vi "RPC Method Measurement_v1_MeasurementService_Measure.vi"(8 "error in (no error)":errorcluster, 10 "Request Data":T4, 11 "gRPC Client in":refnum<class "Measurement_lv_client.lvclass">) -> (0 "error out":errorcluster, 2 "Response Data":T1, 3 "gRPC Client out":refnum<class "Measurement_lv_client.lvclass">)   [LabVIEW 2020, in "Measurement_lv_client.lvlib" / "Measurement_lv_client.lvclass"]
uses:
  Measurement_lv_client.lvclass
  RPC Messages/Measurement_v1_MeasureRequest/Measurement_v1_MeasureRequest_Data.ctl
  RPC Messages/google_protobuf_Any/google_protobuf_Any_Data.ctl
  RPC Messages/Measurement_v1_MeasureResponse/Measurement_v1_MeasureResponse_Data.ctl
  RPC Messages/Measurement_v1_ErrorInformation/Measurement_v1_ErrorInformation_Data.ctl
  Measurement_lv_client.lvclass/Measurement_lv_client.ctl
  fa22ca14-33b2-4bc3-8699-3f27c9b27c9c.vi
  <vilib>/gRPC/LabVIEW gRPC Library/Server API/Server/Get Server DLL Path.vi
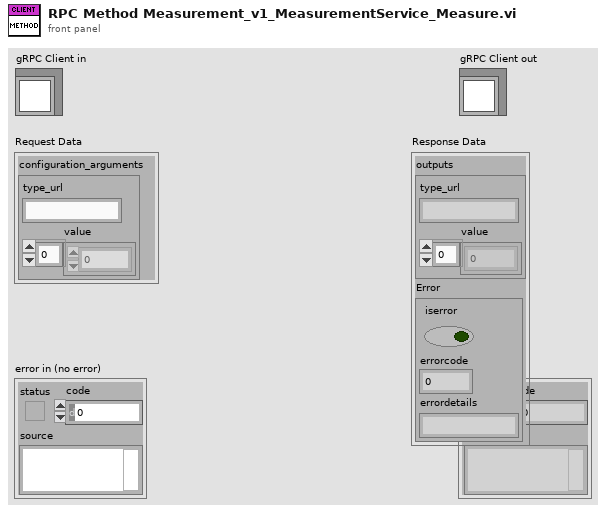
[diagram p1: front panel]
types:
  T1 = typedef "Measurement_lv_client.lvlib/Measurement_lv_client.lvclass/Measurement_v1_MeasureResponse_Data.ctl" = cluster{"outputs":T2, "Error":T3}
  T2 = typedef "Measurement_lv_client.lvlib/Measurement_lv_client.lvclass/google_protobuf_Any_Data.ctl" = cluster{"type_url":string, "value":u8[]}
  T3 = typedef "Measurement_lv_client.lvlib/Measurement_lv_client.lvclass/Measurement_v1_ErrorInformation_Data.ctl" = cluster{"iserror":bool, "errorcode":i32, "errordetails":string}
  T4 = typedef "Measurement_lv_client.lvlib/Measurement_lv_client.lvclass/Measurement_v1_MeasureRequest_Data.ctl" = cluster{"configuration_arguments":T2}
  T5 = typedef "gprc-lvsupport-release.lvlib/grpcId.ctl" = u64
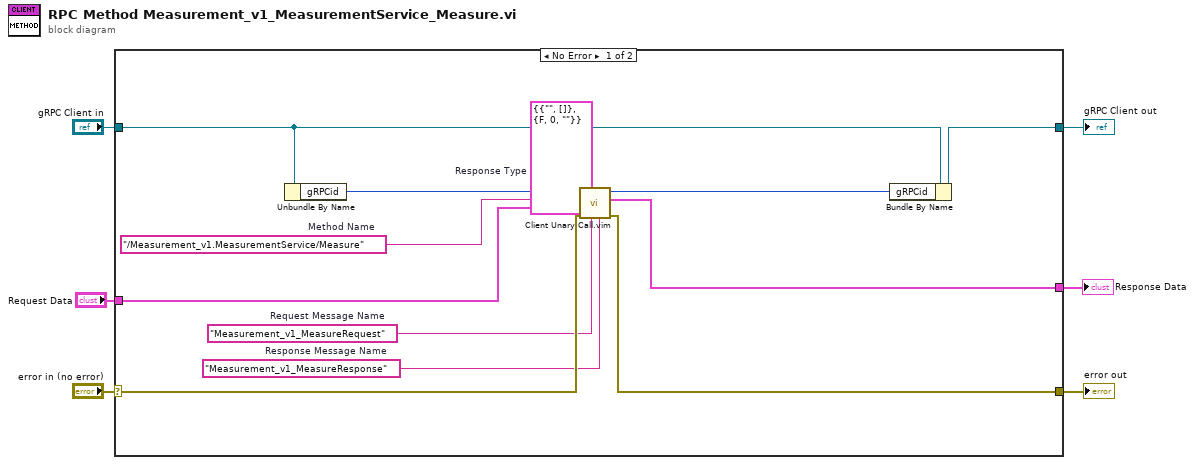
[diagram p0: block diagram]
diagram:
  n1 = case shown="No Error" "error in (no error)" {
    selector: "error in (no error)" -> [w14 w20]
    tunnel: [w13 w20] -> w5
    tunnel: [w15 w19] -> w3
    tunnel: "gRPC Client in" -> [w17 w19]
    tunnel: "Request Data" -> [w11 _]
    tunnel: [w10 _] -> w1
    frame No Error {
      w7 = "Measurement_v1_MeasureResponse"  # Response Message Name
      w8 = "Measurement_v1_MeasureRequest"  # Request Message Name
      w9 = T1 {"outputs"={"type_url"="", "value"=[]}, "Error"={"iserror"=FALSE, "errorcode"=0, "errordetails"=""}}  # Response Type
      w12 = "/Measurement_v1.MeasurementService/Measure"  # Method Name
      n2 = Unbundle By Name(w17) -> ("gRPCid"=w18:T5)
      n3 = call "Client Unary Call.vim"("Response Message Name"=w7, "Request Message Name"=w8, "Response Type"=w9, "error in (no error)"=w14, "Request Data"=w11, "Method Name"=w12, "Client Ref"=w18) -> ("error out"=w13:errorcluster, "Response Data"=w10:T1, "Client Ref Out"=w16:u64)  [unwired: 2 in]
      n4 = Bundle By Name(cluster=w17, "gRPCid"=w16) -> (w15:refnum<class "Measurement_lv_client.lvclass">)
    }
    frame Error {
    }
  }
  "error out" <- w5
  "gRPC Client out" <- w3
  "Response Data" <- w1
